vi "clear_db.vi"() -> ()   [LabVIEW 2010]
uses:
  <vilib>/addons/database/Connection.llb/DB Tools Open Connec (Path).vi
  <vilib>/addons/database/NI_Database_API.lvlib
panel:
  out "tables":string[](array[string])
  out "error out":errorcluster
  in  "connection information":path
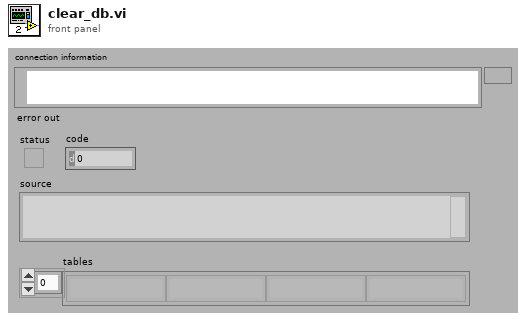
[diagram p1: front panel]
types:
  T1 = typedef "NI_Database_API.lvlib/Conn ObjectReference.ctl" = refnum<k1>
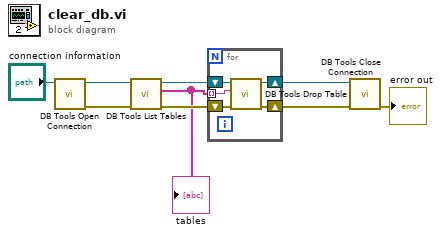
[diagram p0: block diagram]
diagram:
  n1 = call-poly <vilib>:"DB Tools Open Connection.vi"("connection information"="connection information") -> ("error out"=w8:errorcluster, "connection reference"=w9:T1)  [unwired: 7 in]
  n2 = call <vilib>:"DB Tools List Tables.vi"("error in (no error)"=w8, "connection reference"=w9) -> ("error out"=w4:errorcluster, "tables"=w3:string[], "connection reference out"=w7:T1)  [unwired: 3 in]
  "tables" <- w3
  n3 = for {
    shift-right: [w12] -> w5
    shift-left: w4 -> [w11]
    shift-right: [w13] -> w6
    shift-left: w7 -> [w14]
    tunnel: w3 -> [w10] mode=indexing
    n4 = call <vilib>:"DB Tools Drop Table.vi"("error in (no error)"=w11, "table"=w10, "connection reference"=w14) -> ("error out"=w12:errorcluster, "connection reference out"=w13:T1)  [unwired: 5 in]
  }
  n5 = call <vilib>:"DB Tools Close Connection.vi"("error in (no error)"=w5, "connection reference"=w6) -> ("error out"=→"error out":errorcluster)  [unwired: 5 in]
